vi "Read Children Symbol Information.vi"(8 "error in (no error)":errorcluster, 9 "Get all descendents?":bool, 10 "Parent Symbol Name":string, 11 "TwinCAT ADS in":refnum<class "TwinCAT ADS.lvclass">) -> (0 "error out":errorcluster, 1 "Symbols Information":T1[](array[typedef]) {"Type ID" items=["ADST_VOID"=0, "ADST_INT16"=2, "ADST_INT32"=3, "ADST_REAL32"=4, "ADST_REAL64"=5, "ADST_INT8"=16, "ADST_UINT8"=17, "ADST_UINT16"=18, "ADST_UINT32"=19, "ADST_INT64"=20, "ADST_UINT64"=21, "ADST_STRING"=30, "ADST_WSTRING"=31, "ADST_REAL80"=32, "ADST_BIT"=33, "ADST_MAXTYPES"=34, "ADST_BIGTYPE"=65]; "Type Category" items=["Unknown, None"=0, "Primitive"=1, "Alias"=2, "Enum"=3, "Array"=4, "Struct"=5, "FunctionBlock"=6, "Program"=7, "Function"=8, "SubRange"=9, "String"=10, "Bitset"=12, "Pointer"=13, "Union"=14, "Reference"=15, "Interface"=16]}, 3 "TwinCAT ADS out":refnum<class "TwinCAT ADS.lvclass">)   [LabVIEW 2018, in "TwinCAT ADS.lvclass"]
uses:
  TwinCAT ADS.lvclass
  Controls/Symbol Information.ctl
  TwinCAT ADS.lvclass/TwinCAT ADS.ctl
  TwinCAT.Ads
  Get From Symbol Map.vi
  Get From Symbol Map Daemon.vi
  Get Symbol Map.vi
  Format String.vi
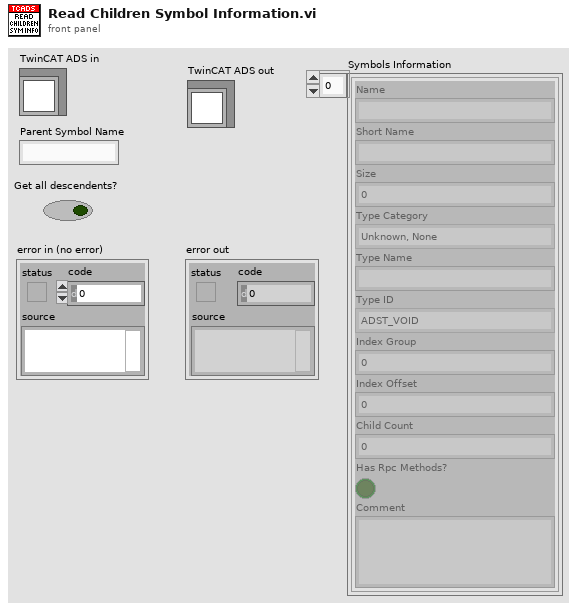
[diagram p1: front panel]
types:
  T1 = typedef "TwinCAT ADS.lvclass/Symbol Information.ctl" = cluster{"Name":string, "Short Name":string, "Size":i32, "Type Category":i32, "Type Name":string, "Type ID":i32, "Index Group":i64, "Index Offset":i64, "Child Count":i32, "Has Rpc Methods?":bool, "Comment":string}
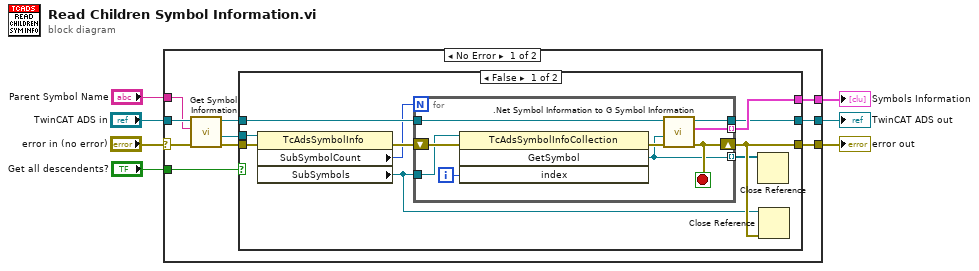
[diagram p0: block diagram]
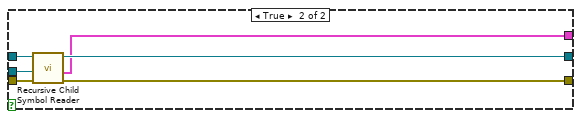
[diagram p2: hidden frame]
diagram:
  n1 = case shown="No Error" "error in (no error)" {
    selector: "error in (no error)" -> [w10 w44]
    tunnel: [w15 w44] -> w2
    tunnel: [w16 w43] -> w1
    tunnel: "TwinCAT ADS in" -> [w13 w43]
    tunnel: "Parent Symbol Name" -> [w9 _]
    tunnel: [w17 _] -> w3
    tunnel: "Get all descendents?" -> [w14 _]
    frame No Error {
      n2 = call "Get Symbol Information.vi"("error in (no error)"=w10, "Symbol Name"=w9, "TwinCAT ADS in"=w13) -> ("error out"=w11:errorcluster, ".NET Symbol Information"=w8:refnum<k24>, "TwinCAT ADS out"=w12:refnum<class "TwinCAT ADS.lvclass">)  [unwired: 6 in]
      n3 = case shown="False" w14 {
        tunnel: w11 -> [w26 w42]
        tunnel: w12 -> [w23 w41]
        tunnel: [w27 w37] -> w17
        tunnel: [w21 w39] -> w16
        tunnel: [w20 w38] -> w15
        tunnel: w8 -> [w24 w40]
        frame False {
          n4 = property class="TcAdsSymbolInfo"(reference=w24, error in=w26) -> (error out=w25:errorcluster, "SubSymbolCount"=w22:i32, "SubSymbols"=w18:refnum<k24>)  [unwired: 1 out]
          n5 = for {
            N: w22 -> [_]
            shift-right: [w29] -> w20
            shift-left: w25 -> [w34]
            tunnel: [w32] -> w27 mode=indexing
            tunnel: w18 -> [w33]
            tunnel: w23 -> [w31]
            tunnel: [w30] -> w21
            tunnel: [w28] -> w19 mode=indexing
            i -> [w35]
            stop <- w29 stop-if-true
            n6 = invoke class="TcAdsSymbolInfoCollection" method="GetSymbol"(reference=w33, error in=w34, "index"=w35) -> (error out=w36:errorcluster, "GetSymbol"=w28:refnum<k24>)  [unwired: 1 in, 2 out]
            n7 = call ".Net Symbol Information to G Symbol Information.vi"("TwinCAT ADS in"=w31, ".NET AdsSymbolInfo"=w28, "error in (no error)"=w36) -> ("TwinCAT ADS out"=w30:refnum<class "TwinCAT ADS.lvclass">, "Symbol Information"=w32:T1, "error out"=w29:errorcluster)  [unwired: 5 in]
          }
          n8 = Close Reference(reference=w19) -> ()  [unwired: 1 in, 1 out]
          n9 = Close Reference(reference=w18, error in (no error)=w20) -> ()  [unwired: 1 out]
        }
        frame True {
          n10 = call "Recursive Child Symbol Reader.vi"("error in (no error)"=w42, ".NET TcAdsSymbolInfo"=w40, "TwinCAT ADS in"=w41) -> ("error out"=w38:errorcluster, "Symbols Information"=w37:T1[], "TwinCAT ADS out"=w39:refnum<class "TwinCAT ADS.lvclass">)  [unwired: 6 in]
        }
      }
    }
    frame Error {
    }
  }
  "error out" <- w2
  "TwinCAT ADS out" <- w1
  "Symbols Information" <- w3
